vi "DriveToXY.vi"(1 "Drive Margin":dbl=2.0, 2 "Steer Margin":dbl=3.0, 5 "X Target":dbl, 7 "Y Target":dbl, 9 "Speed":dbl, 11 "error in":errorcluster) -> (4 "RobotDriveDevRef Out":T1={"DevStatus"={"status"=FALSE, "code"=0, "source"=""}, "Motors[]"=[], "Square Inputs"=FALSE, "Max Output"=1.0, "Isochronous"=FALSE}, 6 "At Target":bool, 15 "error out":errorcluster)   [LabVIEW 2011]
uses:
  <vilib>/Rock Robotics/WPI/RobotDrive/WPI_RobotDriveDevRef.ctl
  <vilib>/Rock Robotics/WPI/MotorControl/WPI_MotorControlDeviceRef.ctl
  <vilib>/Rock Robotics/SystemInterfaces/Typedef/FPGA_TypedefDigitalModule.ctl
  <vilib>/Rock Robotics/SystemInterfaces/DIO/FPGA_DIOPWMChannel.ctl
  <vilib>/Rock Robotics/WPI/PWM/WPI_PWMDeadband.ctl
  <vilib>/Rock Robotics/WPI/CAN/Jaguar/SubVIs/WPI_CANJaguar_ControlMode.ctl
  <vilib>/Rock Robotics/WPI/PWM/WPI_PWMTransform_ConPane.ctl
  Robot Global Data.vi
  <vilib>/addons/control/pid/NI_PID_pid.lvlib
panel:
  in  "Drive PID gains":T9={"proportional gain (Kc)"=0.05, "integral time (Ti, min)"=0.0, "derivative time (Td, min)"=0.0} {"derivative time (Td, min)" format="%.3f"; "integral time (Ti, min)" format="%.3f"; "proportional gain (Kc)" format="%.3f"}
  in  "Steer PID gains":T9={"proportional gain (Kc)"=0.02, "integral time (Ti, min)"=0.01, "derivative time (Td, min)"=0.002} {"derivative time (Td, min)" format="%#.7g"; "integral time (Ti, min)" format="%#.6g"; "proportional gain (Kc)" format="%#.6g"}
  in  "Steering Saturation":dbl=1.0
  # "0.02"
  # "0.03\n0\n0"
  # "0.05"
  # "0.01"
  # "0.002"
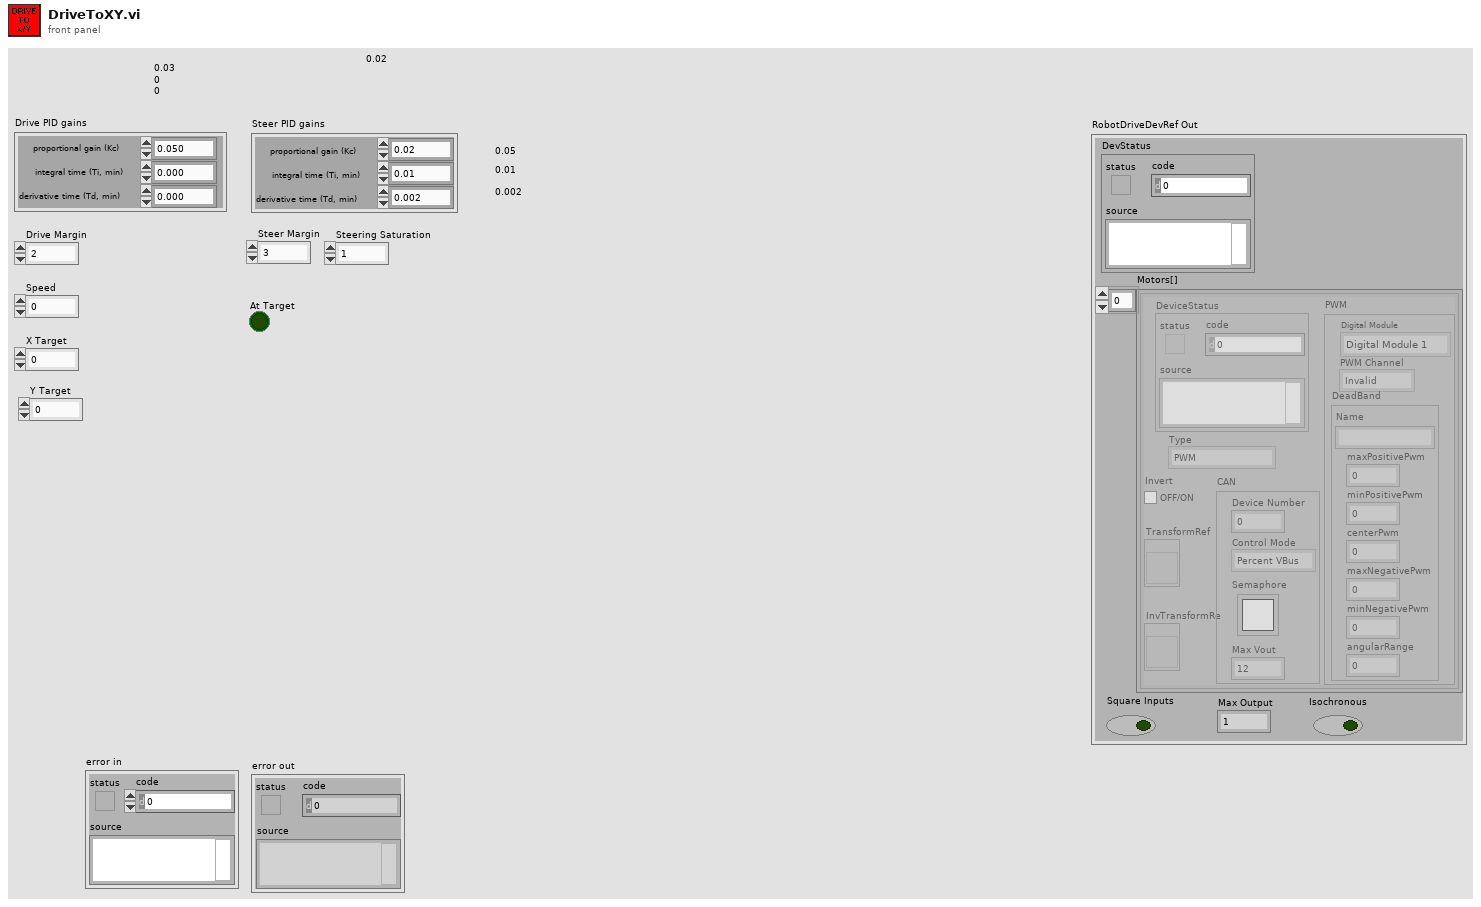
[diagram p1: front panel]
types:
  T1 = typedef "WPI_RobotDriveDevRef.ctl" = cluster{"DevStatus":errorcluster, "Motors[]":T2[], "Square Inputs":bool, "Max Output":dbl, "Isochronous":bool}
  T2 = typedef "WPI_MotorControlDeviceRef.ctl" = cluster{"DeviceStatus":errorcluster, "Type":enum16{"PWM", "CAN"}, "PWM":cluster{"Digital Module":T3, "PWM Channel":T4, "DeadBand":T5}, "CAN":cluster{"Device Number":u8, "Control Mode":T6, "Semaphore":T7, "Max Vout":dbl}, "Invert":bool, "TransformRef":T8, "InvTransformRef":T8}
  T3 = typedef "FPGA_TypedefDigitalModule.ctl" = enum16{"Digital Module 1", "Digital Module 2"}
  T4 = typedef "FPGA_DIOPWMChannel.ctl" = enum8{"PWM 1", "PWM 2", "PWM 3", "PWM 4", "PWM 5", "PWM 6", "PWM 7", "PWM 8", "PWM 9", "PWM 10", "Invalid"}
  T5 = typedef "WPI_PWMDeadband.ctl" = cluster{"Name":string, "maxPositivePwm":i32, "minPositivePwm":i32, "centerPwm":i32, "maxNegativePwm":i32, "minNegativePwm":i32, "angularRange":u16}
  T6 = typedef "WPI_CANJaguar_ControlMode.ctl" = enum8{"Percent VBus", "Current", "Speed", "Position", "Voltage"}
  T7 = typedef "Semaphore RefNum" = refnum<k1>
  T8 = typedef "WPI_PWMTransform_ConPane.ctl" = refnum<vi>
  T9 = cluster{"proportional gain (Kc)":dbl, "integral time (Ti, min)":dbl, "derivative time (Td, min)":dbl}
  T10 = typedef "Position Typedef.ctl" = cluster{"X":dbl, "Y":dbl, "Heading":dbl}
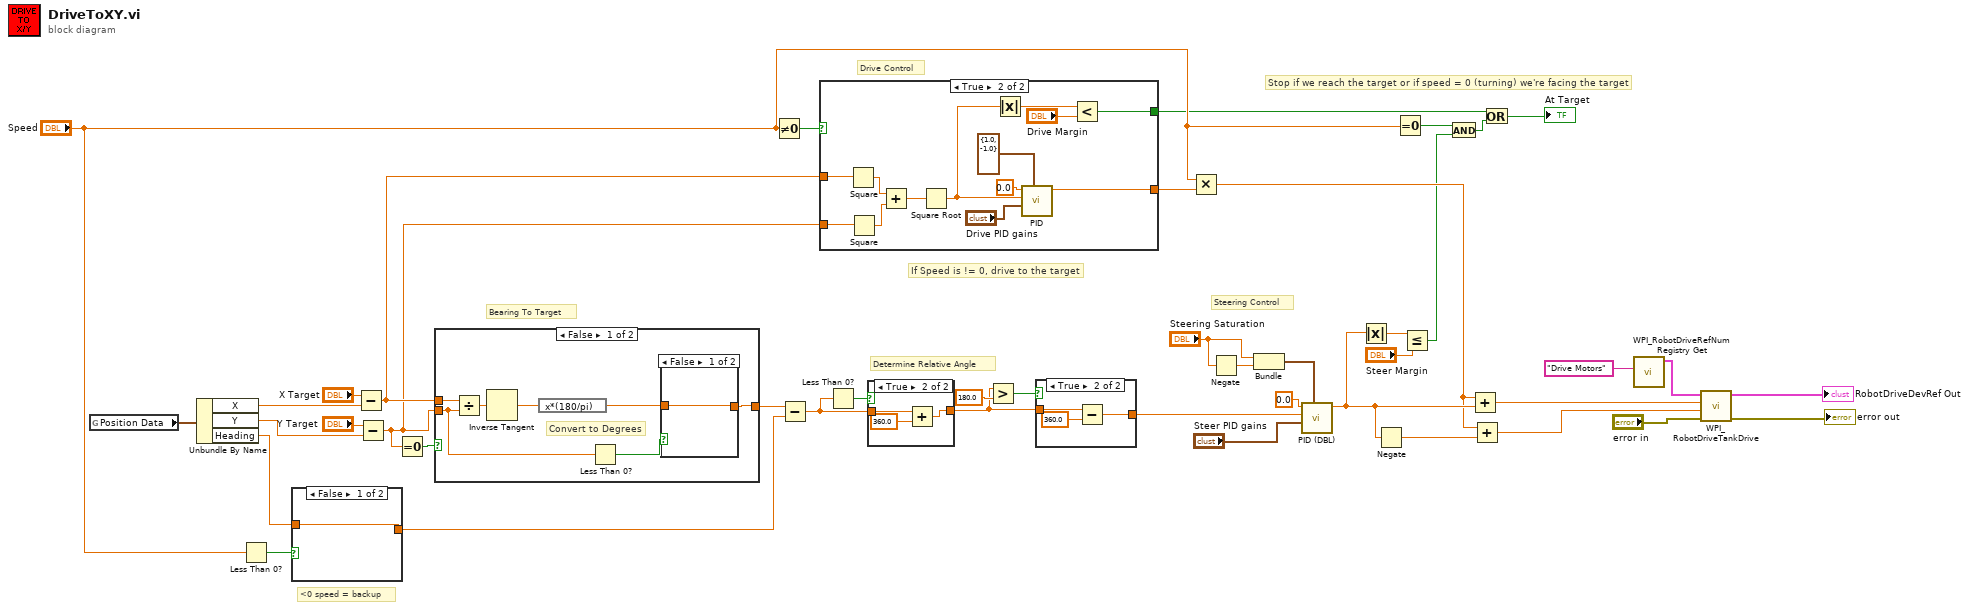
[diagram p0: block diagram]
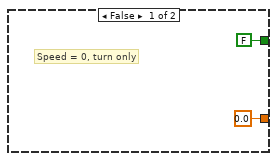
[diagram p2: hidden frame]
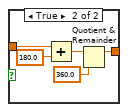
[diagram p5: hidden frame]
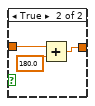
[diagram p6: hidden frame]
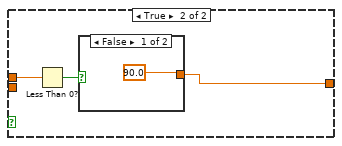
[diagram p7: hidden frame]
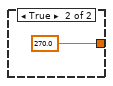
[diagram p8: hidden frame]
diagram:
  # "Stop if we reach the target or if speed = 0 (turning) we're facing the target"
  # "Drive Control"
  # "If Speed is != 0, drive to the target"
  # "Steering Control"
  # "Determine Relative Angle"
  # "Bearing To Target"
  # "<0 speed = backup"
  n1 = global read "Robot Global Data.vi" "Position Data"() -> (w43:T10)
  n2 = Unbundle By Name(w43) -> ("X"=w22:dbl, "Y"=w21:dbl, "Heading"=w39:dbl)
  n3 = Less Than 0?(x="Speed") -> (x < 0?=w36:bool)
  n4 = case shown="False" w36 {
    tunnel: w39 -> [w44 w46]
    tunnel: [w44 w45] -> w37
    frame False {
    }
    frame True {
      n5 = Add(x=w46, y=180.0) -> (x+y=w48:dbl)
      n6 = Quotient & Remainder(x=w48, y=360.0) -> (x-y*floor(x/y)=w45:dbl)  [unwired: 1 out]
    }
  }
  n7 = Subtract(x="X Target", y=w22) -> (x-y=w20:dbl)
  n8 = Subtract(x="Y Target", y=w21) -> (x-y=w19:dbl)
  n9 = Equal To 0?(x=w19) -> (x = 0?=w40:bool)
  n10 = case shown="False" w40 {
    tunnel: w20 -> [w56 w62]
    tunnel: [w51 w61] -> w38
    tunnel: w19 -> [w53 _]
    frame False {
      # "Convert to Degrees"
      n11 = Divide(x=w56, y=w53) -> (x/y=w54:dbl)
      n12 = Inverse Tangent(1:w54) -> (0:w55:dbl)
      n13 = expression code="x*(180/pi)"(w55) -> (w50:dbl)
      n14 = Less Than 0?(x=w53) -> (x < 0?=w52:bool)
      n15 = case shown="False" w52 {
        tunnel: [w57 w60] -> w51
        tunnel: w50 -> [w57 w59]
        frame False {
        }
        frame True {
          n16 = Add(x=w59, y=180.0) -> (x+y=w60:dbl)
        }
      }
    }
    frame True {
      n17 = Less Than 0?(x=w62) -> (x < 0?=w63:bool)
      n18 = case shown="False" w63 {
        tunnel: [90.0 ("y") 270.0 ("y")] -> w61
        frame False {
        }
        frame True {
        }
      }
    }
  }
  n19 = Not Equal To 0?(x="Speed") -> (x != 0?=w16:bool)
  n20 = Subtract(x=w38, y=w37) -> (x-y=w31:dbl)
  n21 = case shown="True" w16 {
    tunnel: w20 -> [_ w71]
    tunnel: w19 -> [_ w70]
    tunnel: [FALSE w69] -> w10
    tunnel: [0.0 ("output") w68] -> w15
    frame False {
      # "Speed = 0, turn only"
    }
    frame True {
      n22 = Square(x=w71) -> (x^2=w78:dbl)
      n23 = Square(x=w70) -> (x^2=w77:dbl)
      n24 = Add(x=w78, y=w77) -> (x+y=w76:dbl)
      n25 = Square Root(x=w76) -> (sqrt(x)=w73:dbl)
      n26 = Absolute Value(x=w73) -> (abs(x)=w75:dbl)
      n27 = call-poly <vilib>:"PID.vi"("output range"=cluster{"output high":dbl, "output low":dbl} {"output high"=1.0, "output low"=-1.0}, "PID gains"="Drive PID gains", "process variable"=w73, "setpoint"=0.0 ("y")) -> ("output"=w68:dbl)  [unwired: 2 in, 5 out]
      n28 = Less?(x=w75, y="Drive Margin") -> (x < y?=w69:bool)
    }
  }
  n29 = Less Than 0?(x=w31) -> (x < 0?=w33:bool)
  n30 = case shown="True" w33 {
    tunnel: w31 -> [w81 w83]
    tunnel: [w81 w82] -> w32
    frame False {
    }
    frame True {
      n31 = Add(x=w83, y=360.0) -> (x+y=w82:dbl)
    }
  }
  n32 = Greater?(x=w32, y=180.0) -> (0:w34:bool)
  n33 = case shown="True" w34 {
    tunnel: w32 -> [w85 w88]
    tunnel: [w85 w87] -> w26
    frame False {
    }
    frame True {
      n34 = Subtract(x=w88, y=360.0) -> (x-y=w87:dbl)
    }
  }
  n35 = Multiply(x="Speed", y=w15) -> (x*y=w12:dbl)
  n36 = Negate(x="Steering Saturation") -> (-x=w29:dbl)
  n37 = Bundle("Steering Saturation"="Steering Saturation", w29) -> (w28:cluster{"Steering Saturation":dbl, dbl})  [unwired: 1 out]
  n38 = call <vilib>:"PID (DBL).vi"("output range"=w28, "PID gains"="Steer PID gains", "process variable"=w26, "setpoint"=0.0) -> ("output"=w14:dbl)  [unwired: 2 in, 5 out]
  n39 = Absolute Value(x=w14) -> (abs(x)=w18:dbl)
  n40 = Negate(x=w14) -> (-x=w13:dbl)
  n41 = Equal To 0?(x="Speed") -> (x = 0?=w8:bool)
  n42 = Less Or Equal?(x=w18, y="Steer Margin") -> (x <= y?=w7:bool)
  n43 = And(x=w8, y=w7) -> (x .and. y?=w9:bool)
  n44 = Add(x=w12, y=w14) -> (x+y=w24:dbl)
  n45 = Add(x=w12, y=w13) -> (x+y=w23:dbl)
  n46 = Or(x=w10, y=w9) -> (x .or. y?=→"At Target":bool)
  n47 = call <vilib>:"WPI_RobotDriveRefNum Registry Get.vi"("refnum name"="Drive Motors") -> ("RobotDriveDevRef"=w3:T1)  [unwired: 1 in, 9 out]
  n48 = call <vilib>:"WPI_RobotDriveTankDrive.vi"("error in (no error)"="error in", "Right axis value"=w23, "Left axis value"=w24, "RobotDriveDevRef"=w3) -> ("error out"=→"error out":errorcluster, "RobotDriveDevRef"=→"RobotDriveDevRef Out":T1)  [unwired: 6 in]
